vi "MotoSignalSet.vi"(1 "CAN64B簇":cluster{"时间(s)":dbl[], "Data64Bits(u64)":u64[]}, 2 "信号格式簇":T1) -> (6 "信号":cluster{"时间(s)":dbl[], "数据":dbl[]})   [LabVIEW 2015]
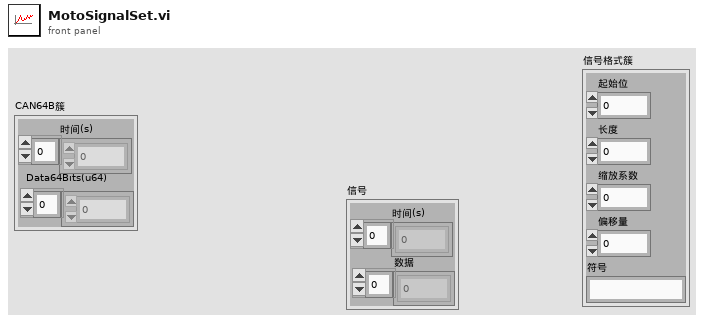
[diagram p1: front panel]
types:
  T1 = cluster{"起始位":u8, "长度":u8, "缩放系数":dbl, "偏移量":dbl, "符号":string}
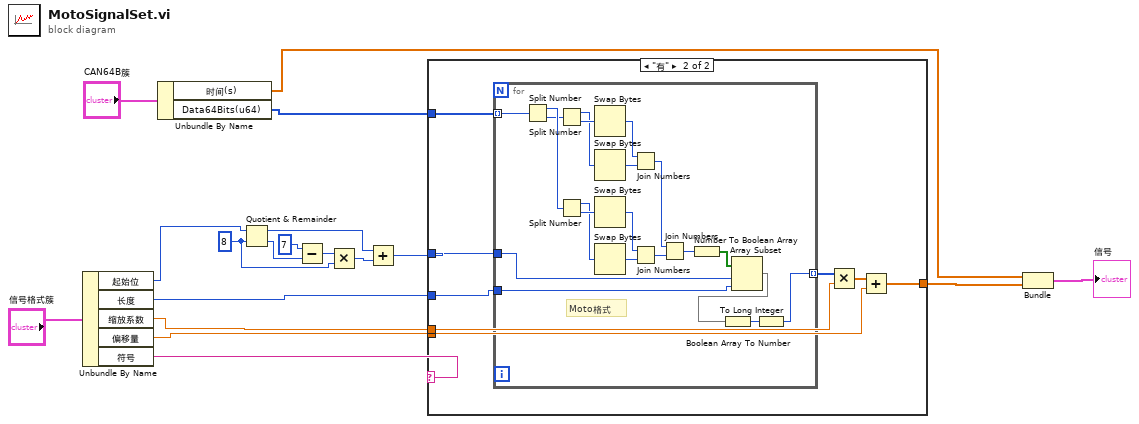
[diagram p0: block diagram]
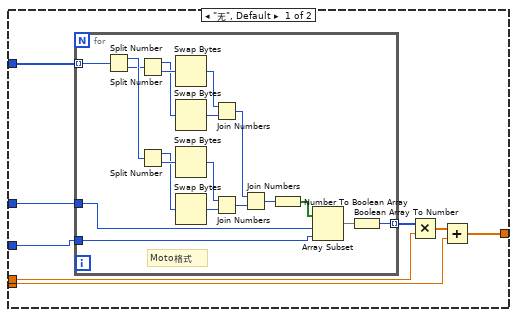
[diagram p2: hidden frame]
diagram:
  w11 = 8
  n1 = Unbundle By Name("信号格式簇") -> ("起始位"=w2:u8, "长度"=w3:u8, "缩放系数"=w4:dbl, "偏移量"=w5:dbl, "符号"=w1:string)
  n2 = Unbundle By Name("CAN64B簇") -> ("时间(s)"=w7:dbl[], "Data64Bits(u64)"=w8:u64[])
  n3 = Quotient & Remainder(x=w2, y=w11) -> (x-y*floor(x/y)=w16:i32, floor(x/y)=w14:i32)
  n4 = Subtract(x=7, y=w14) -> (x-y=w15:i32)
  n5 = Multiply(x=w15, y=w11) -> (x*y=w13:i32)
  n6 = Add(x=w16, y=w13) -> (x+y=w10:i32)
  n7 = case shown="\"有\"" w1 {
    tunnel: [w26 w53] -> w18
    tunnel: w10 -> [w23 w50]
    tunnel: w8 -> [w22 w49]
    tunnel: w5 -> [w21 w48]
    tunnel: w4 -> [w20 w47]
    tunnel: w3 -> [w19 w46]
    frame "无", Default {
      n8 = for {
        tunnel: w22 -> [w42] mode=indexing
        tunnel: w19 -> [w45]
        tunnel: [w44] -> w24 mode=indexing
        tunnel: w23 -> [w27]
        # "Moto格式"
        n9 = Split Number(x=w42) -> (hi(x)=w41:u32, lo(x)=w40:u32)
        n10 = Split Number(x=w40) -> (hi(x)=w38:u16, lo(x)=w39:u16)
        n11 = Split Number(x=w41) -> (hi(x)=w36:u16, lo(x)=w37:u16)
        n12 = Swap Bytes(anything=w39) -> (byte swapped=w33:u16)
        n13 = Swap Bytes(anything=w38) -> (byte swapped=w32:u16)
        n14 = Swap Bytes(anything=w37) -> (byte swapped=w34:u16)
        n15 = Swap Bytes(anything=w36) -> (byte swapped=w35:u16)
        n16 = Join Numbers(hi=w33, lo=w32) -> ((hi.lo)=w30:u32)
        n17 = Join Numbers(hi=w34, lo=w35) -> ((hi.lo)=w31:u32)
        n18 = Join Numbers(hi=w30, lo=w31) -> ((hi.lo)=w29:u64)
        n19 = Number To Boolean Array(number=w29) -> (Boolean array=w28:bool[])
        n20 = Array Subset(array=w28, index=w27, length=w45) -> (w43:bool[])
        n21 = Boolean Array To Number(Boolean array=w43) -> (number=w44:u32)
      }
      n22 = Multiply(x=w24, y=w20) -> (x*y=w25:dbl[])
      n23 = Add(x=w25, y=w21) -> (x+y=w26:dbl[])
    }
    frame "有" {
      n24 = for {
        tunnel: w49 -> [w71] mode=indexing
        tunnel: w46 -> [w73]
        tunnel: [w54] -> w51 mode=indexing
        tunnel: w50 -> [w56]
        # "Moto格式"
        n25 = Split Number(x=w71) -> (hi(x)=w70:u32, lo(x)=w69:u32)
        n26 = Split Number(x=w69) -> (hi(x)=w67:u16, lo(x)=w68:u16)
        n27 = Split Number(x=w70) -> (hi(x)=w65:u16, lo(x)=w66:u16)
        n28 = Swap Bytes(anything=w68) -> (byte swapped=w62:u16)
        n29 = Swap Bytes(anything=w67) -> (byte swapped=w61:u16)
        n30 = Swap Bytes(anything=w66) -> (byte swapped=w63:u16)
        n31 = Swap Bytes(anything=w65) -> (byte swapped=w64:u16)
        n32 = Join Numbers(hi=w62, lo=w61) -> ((hi.lo)=w59:u32)
        n33 = Join Numbers(hi=w63, lo=w64) -> ((hi.lo)=w60:u32)
        n34 = Join Numbers(hi=w59, lo=w60) -> ((hi.lo)=w58:u64)
        n35 = Number To Boolean Array(number=w58) -> (Boolean array=w57:bool[])
        n36 = Array Subset(array=w57, index=w56, length=w73) -> (w72:bool[])
        n37 = Boolean Array To Number(Boolean array=w72) -> (number=w55:u32)
        n38 = To Long Integer(number=w55) -> (32bit integer=w54:i32)
      }
      n39 = Multiply(x=w51, y=w47) -> (x*y=w52:dbl[])
      n40 = Add(x=w52, y=w48) -> (x+y=w53:dbl[])
    }
  }
  n41 = Bundle("时间(s)"=w7, w18) -> (→"信号":cluster{"时间(s)":dbl[], dbl[]})  [unwired: 1 in]
